vi "Initialize.vi"(8 "error in":errorcluster, 11 "Serial Master in":refnum<class "Serial Data Unit.lvclass">) -> (0 "error out":errorcluster, 3 "Serial Master out":refnum<class "Serial Data Unit.lvclass">)   [LabVIEW 2021, in "Serial Data Unit.lvclass"]
doc: "This provides an interface for the master to open a connection to the slave."
uses:
  Serial Data Unit.lvclass
  Serial Data Unit.lvclass/Serial Data Unit.ctl
  Network Interface/Serial Interface/SSC/Serial Shared Components.lvlib
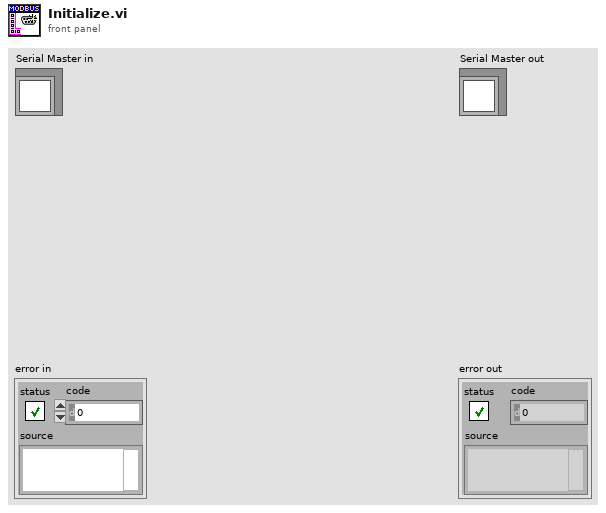
[diagram p1: front panel]
types:
  T1 = enum16{"None", "XON/XOFF", "RTS/CTS", "XON/XOFF & RTS/CTS", "DTR/DSR", "XON/XOFF & DTR/DSR"}
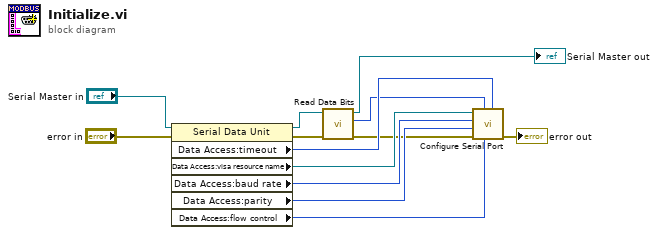
[diagram p0: block diagram]
diagram:
  n1 = property class="Serial Data Unit"(reference="Serial Master in", error in="error in") -> (reference out=w1:refnum<class "Serial Data Unit.lvclass">, error out=w6:errorcluster, "Data Access:timeout"=w7:u32, "Data Access:visa resource name"=w13:refnum<visa-resource-name>, "Data Access:baud rate"=w12:u32, "Data Access:parity"=w11:enum16{"None", "Odd", "Even", "Mark", "Space"}, "Data Access:flow control"=w10:T1)
  n2 = call-dynamic "Read Data Bits.vi"("error in (no error)"=w6, "Serial Data Unit in"=w1) -> ("error out"=w5:errorcluster, "data bits"=w3:u16, "Serial Data Unit out"=→"Serial Master out":refnum<class "Serial Data Unit.lvclass">)  [unwired: 7 in]
  n3 = call "Configure Serial Port.vi"("Timeout"=w7, "Flow Control"=w10, "data bits"=w3, "error in (no error)"=w5, "Parity"=w11, "Baud Rate"=w12, "VISA Refnum in"=w13) -> ("error out"=→"error out":errorcluster)  [unwired: 4 in]
